vi "replaceReDoneTriples.vi"(8 "error in (no error)":errorcluster, 11 "Utilities in":refnum<class "Utilities.lvclass">) -> (0 "error out":errorcluster, 3 "Utilities out":refnum<class "Utilities.lvclass">)   [LabVIEW 2020, in "Utilities.lvclass"]
uses:
  Utilities.lvclass
panel:
  in  "destination path":path=path "C:/Users/RoboIme/git/sslview/Util/Farias2.csv"
  in  "mean_values_header (default)":string[](array[string])=["V0", "Vf", "V_sent", "D", "dt", "triple_id", "considered_samples"]
  out "originalMean":dbl[][](array[numeric])
  out "originalstd":dbl[][](array[numeric])
  out "meanWithReDoneReplaced":dbl[][](array[numeric])
  out "stdWithReDoneReplaced":dbl[][](array[numeric])
  in  "original mean ReDone":path=path "C:/Users/RoboIme/git/sslview/Util/Farias2.csv"
  in  "std path ReDone":path=path "C:/Users/RoboIme/git/sslview/Util/Farias2.csv"
  in  "original mean path":path=path "C:/Users/RoboIme/git/sslview/Util/Farias2.csv"
  in  "origianal std path":path=path "C:/Users/RoboIme/git/sslview/Util/Farias2.csv"
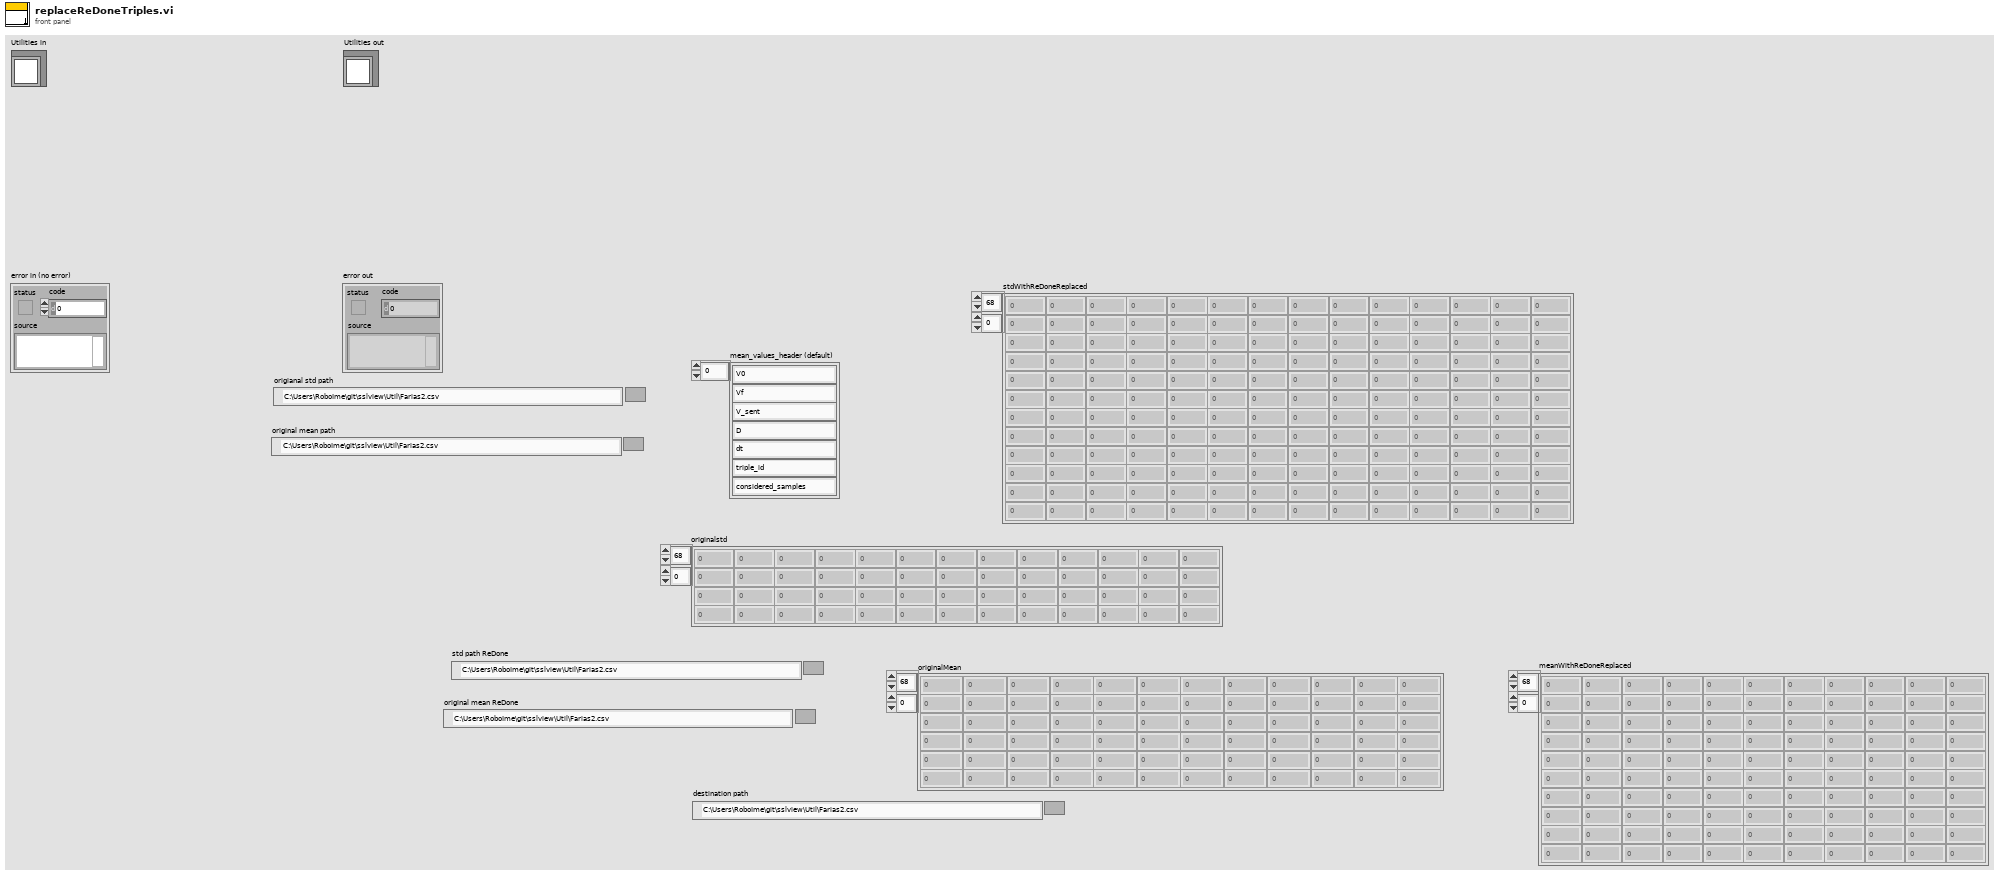
[diagram p1: front panel]
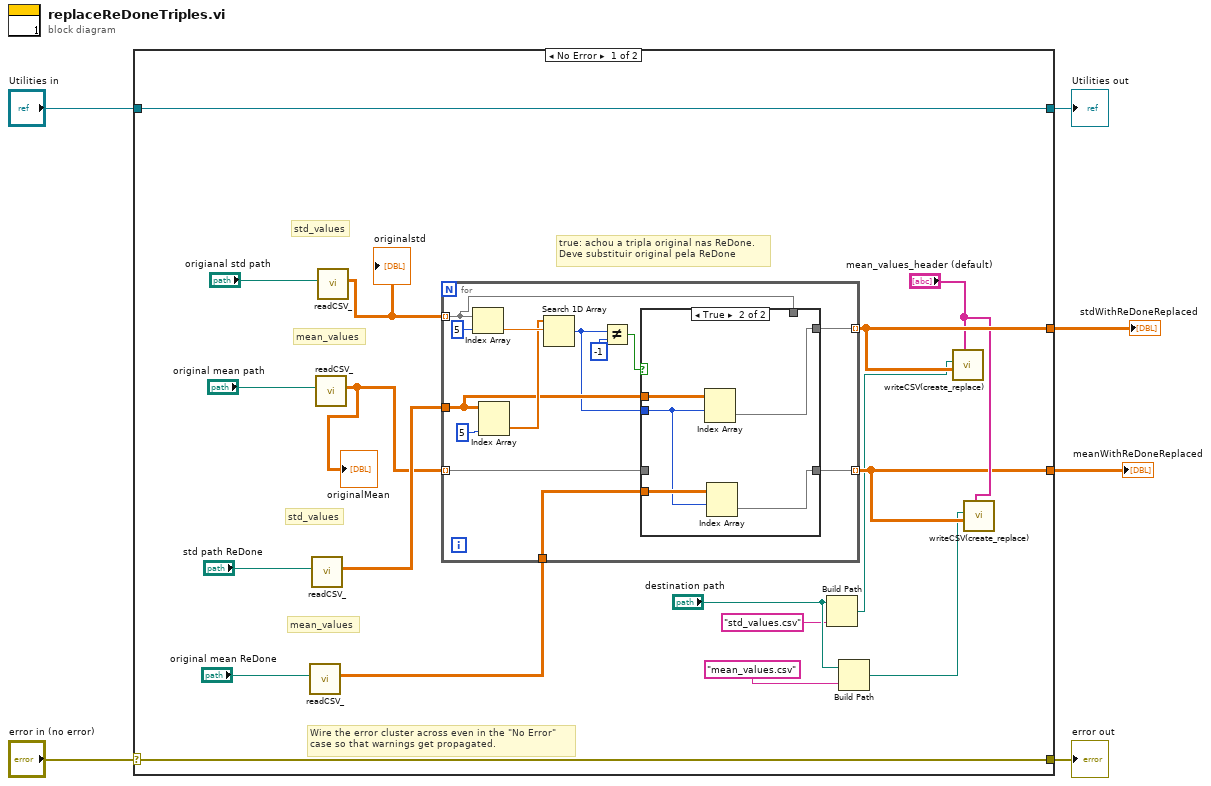
[diagram p0: block diagram]
diagram:
  n1 = case shown="No Error" "error in (no error)" {
    selector: "error in (no error)" -> [w23 w46]
    tunnel: [w23 w46] -> w5
    tunnel: [w24 w45] -> w3
    tunnel: "Utilities in" -> [w24 w45]
    tunnel: [w14 _] -> w2
    tunnel: [w12 _] -> w1
    frame No Error {
      # "true: achou a tripla original nas ReDone.\nDeve substituir original pela ReDone"
      # "mean_values"
      # "std_values"
      # "mean_values"
      # "std_values"
      # "Wire the error cluster across even in the \"No Error\"\ncase so that warnings get propagated."
      n2 = call "readCSV_.vi"("file path (use dialog)"="original mean ReDone") -> ("array"=w16:dbl[][])  [unwired: 8 in, 2 out]
      n3 = call "readCSV_.vi"("file path (use dialog)"="std path ReDone") -> ("array"=w17:dbl[][])  [unwired: 8 in, 2 out]
      n4 = call "readCSV_.vi"("file path (use dialog)"="original mean path") -> ("array"=w15:dbl[][])  [unwired: 8 in, 2 out]
      "originalMean" <- w15
      n5 = call "readCSV_.vi"("file path (use dialog)"="origianal std path") -> ("array"=w18:dbl[][])  [unwired: 8 in, 2 out]
      "originalstd" <- w18
      n6 = for {
        tunnel: w18 -> [w32] mode=indexing
        tunnel: w15 -> [w29] mode=indexing
        tunnel: w17 -> [w27]
        tunnel: [w31] -> w14 mode=indexing
        tunnel: [w28] -> w12 mode=indexing
        tunnel: w16 -> [w25]
        n7 = Index Array(array=w32, index=5) -> (element=w36:dbl)
        n8 = Index Array(array=w27, index (col)=5 ("index")) -> (element=w30:dbl[])  [unwired: 1 in]
        n9 = Search 1D Array(1D array=w30, element=w36) -> (index of element=w26:i32)  [unwired: 1 in]
        n10 = Not Equal?(x=w26, y=-1) -> (x != y?=w33:bool)
        n11 = case shown="True" w33 {
          tunnel: [w39 w43] -> w31
          tunnel: w32 -> [w39 _]
          tunnel: [w38 w40] -> w28
          tunnel: w29 -> [w38 _]
          tunnel: w27 -> [_ w44]
          tunnel: w26 -> [_ w41]
          tunnel: w25 -> [_ w42]
          frame False {
          }
          frame True {
            n12 = Index Array(array=w44, index (row)=w41) -> (element=w43:dbl[])  [unwired: 1 in]
            n13 = Index Array(array=w42, index (row)=w41) -> (element=w40:dbl[])  [unwired: 1 in]
          }
        }
      }
      n14 = Build Path(base path="destination path", name or relative path="std_values.csv") -> (appended path=w8:path)
      n15 = Build Path(base path="destination path", name or relative path="mean_values.csv") -> (appended path=w7:path)
      n16 = call "writeCSV(create_replace).vi"("Header"="mean_values_header (default)", "Array"=w14, "file path (use dialog)"=w8) -> ()  [unwired: 7 in, 2 out]
      n17 = call "writeCSV(create_replace).vi"("Header"="mean_values_header (default)", "Array"=w12, "file path (use dialog)"=w7) -> ()  [unwired: 7 in, 2 out]
    }
    frame Error {
    }
  }
  "error out" <- w5
  "Utilities out" <- w3
  "stdWithReDoneReplaced" <- w2
  "meanWithReDoneReplaced" <- w1
